vi "delete module from engine.vi"(8 "error in":errorcluster, 10 "module ID":string, 11 "engine configuration in":refnum<class "engine configuration.lvclass">) -> (0 "error out":errorcluster, 3 "engine configuration out":refnum<class "engine configuration.lvclass">)   [LabVIEW 2013, in "engine configuration.lvclass"]
uses:
  engine configuration.lvclass
  engine configuration.lvclass/engine configuration.ctl
  <vilib>/NI/Tag Bus/tag/tag descriptor.lvclass
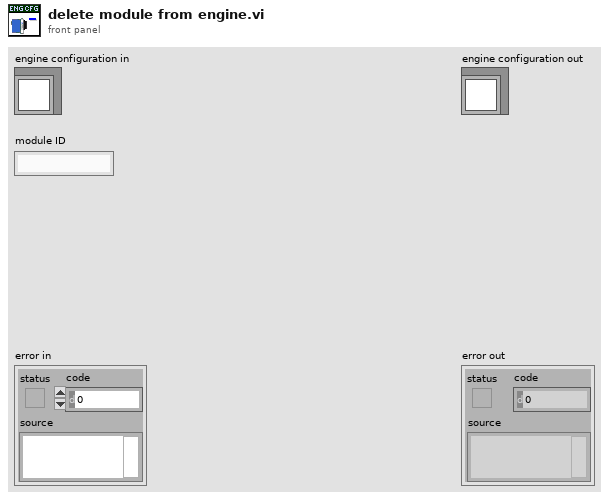
[diagram p1: front panel]
types:
  T1 = typedef "engine configuration.lvclass/Tag Info.ctl" = cluster{"Tag":refnum<class "tag descriptor.lvclass">, "Writer":string, "Readers":string[], "Owning ID":string}
  T2 = typedef "engine configuration.lvclass/Module Mappings.ctl" = cluster{"Owning ID":string, "Input Mappings":T3[], "Process Parameter Mappings":T3[], "Process Results Mappings":T3[], "Output Mappings":T3[]}
  T3 = typedef "tag bus.lvlib/data table.lvlib/mapping specification.ctl" = cluster{"data type":T4, "mappings":T5[]}
  T4 = typedef "tag bus.lvlib/tag descriptor.lvclass/Data Type.ctl" = enum16{"Double", "Single", "I64", "I32", "I16", "I8", "U64", "U32", "U16", "U8", "Boolean", "String", "Array of Double", "Array of Single", "Array of I64", "Array of I32", "Array of I16", "Array of I8", "Array of U64", "Array of U32", "Array of U16", "Array of U8", "Array of Boolean", "Array of String"}
  T5 = typedef "tag bus.lvlib/data table.lvlib/mapping.ctl" = cluster{"sink name":string, "source name":string}
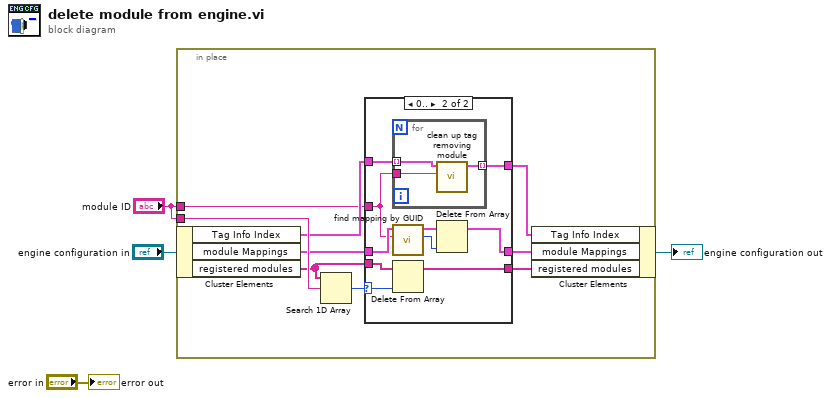
[diagram p0: block diagram]
diagram:
  n1 = in-place {
    in-place-border: "module ID" -> [w13]
    in-place-border: "module ID" -> [w5]
    n2 = in-place-cluster #1("engine configuration in") -> ("Tag Info Index"=w8:T1[], "module Mappings"=w7:T2[], "registered modules"=w12:string[])
    n3 = Search 1D Array(1D array=w12, element=w13) -> (index of element=w10:i32)  [unwired: 1 in]
    n4 = case shown="0.." w10 {
      selector: w10 -> [_ w24]
      tunnel: w12 -> [w14 w26]
      tunnel: [w14 w25] -> w11
      tunnel: [w16 w22] -> w9
      tunnel: w8 -> [w16 w23]
      tunnel: w7 -> [w15 w21]
      tunnel: [w15 w17] -> w6
      tunnel: w5 -> [_ w20]
      frame ..-1 {
      }
      frame 0.. {
        n5 = for {
          tunnel: w23 -> [w29] mode=indexing
          tunnel: [w28] -> w22 mode=indexing
          tunnel: w20 -> [w27]
          n6 = call "clean up tag removing module.vi"("module ID"=w27, "Tag Info in"=w29) -> ("Tag Info out"=w28:T1)  [unwired: 9 in]
        }
        n7 = call "find mapping by GUID.vi"("owner ID"=w20, "module Mappings"=w21) -> ("index"=w18:i32, "module Mappings out"=w19:T2[])  [unwired: 8 in]
        n8 = Delete From Array(array=w26, index=w24) -> (array with subset deleted=w25:string[])  [unwired: 1 in, 1 out]
        n9 = Delete From Array(array=w19, index=w18) -> (array with subset deleted=w17:T2[])  [unwired: 1 in, 1 out]
      }
    }
    n10 = in-place-cluster #1("Tag Info Index"=w9, "module Mappings"=w6, "registered modules"=w11) -> (→"engine configuration out":refnum<class "engine configuration.lvclass">)
  }
  "error out" <- "error in"
